vi "FreqC.Open Session.vi"(8 "error In":errorcluster, 11 "VISA resource name":refnum<visa-resource-name>) -> (0 "error out":errorcluster, 3 "FreqC Session out":T1)   [LabVIEW 2018]
uses:
  typedefs/FreqC.Session.ctl
  <instrlib>/Agilent 532XX Series/Public/Configure/Configure Channel (Basic).vi
  <instrlib>/Agilent 532XX Series/Public/Configure/Configure Channel (Voltage Range).vi
  <instrlib>/Agilent 532XX Series/Public/Configure/Configure Channel (Slop).vi
  <instrlib>/Agilent 532XX Series/Public/Configure/Configure Channel (Threshold Voltage).vi
  <instrlib>/Agilent 532XX Series/Public/Configure/Measurement/Configure Measurement (Totalize Timed).vi
  <instrlib>/Agilent 532XX Series/Agilent 532XX Series.lvlib
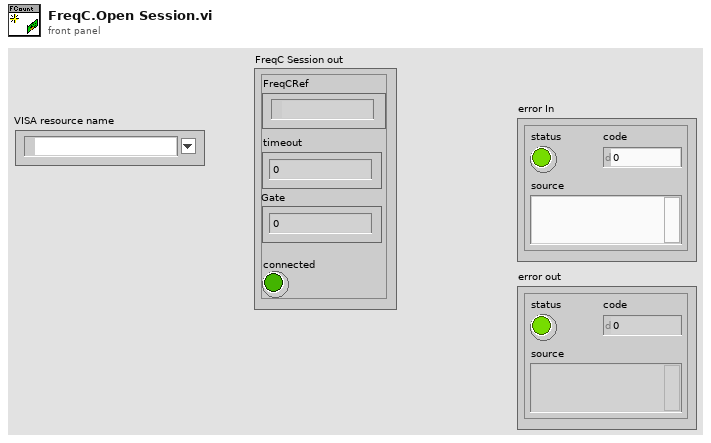
[diagram p1: front panel]
types:
  T1 = typedef "FreqC.Session.ctl" = cluster{"FreqCRef":refnum<visa-resource-name>, "timeout":dbl, "Gate":dbl, "connected":bool}
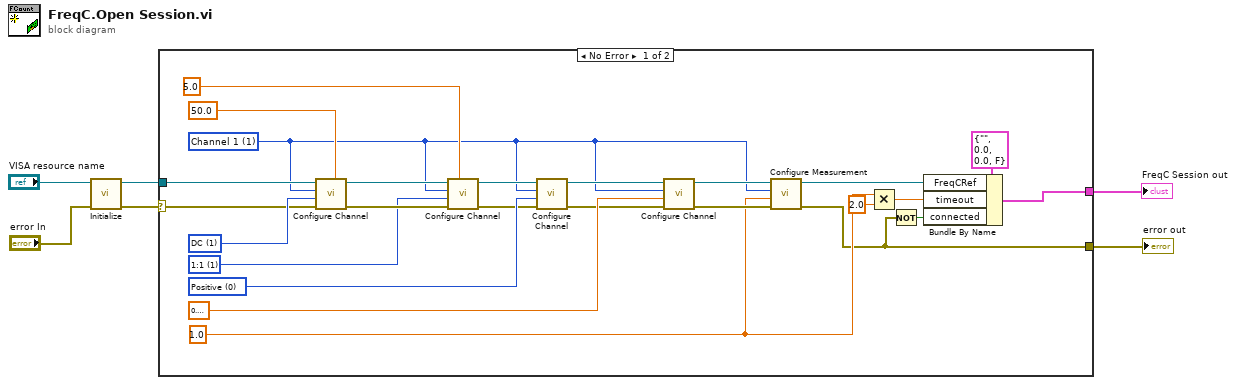
[diagram p0: block diagram]
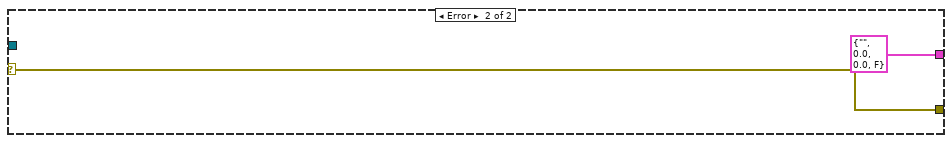
[diagram p2: hidden frame]
diagram:
  n1 = call <instrlib>:"Initialize.vi"("error in (no error)"="error In", "VISA resource name"="VISA resource name") -> ("error out"=w1:errorcluster, "VISA resource name out"=w6:refnum<visa-resource-name>)  [unwired: 8 in]
  n2 = case shown="No Error" w1 {
    selector: w1 -> [w12 w33]
    tunnel: w6 -> [w31 _]
    tunnel: [w7 w33] -> w3
    tunnel: [w13 T1 {"FreqCRef"="", "timeout"=0.0, "Gate"=0.0, "connected"=FALSE} ("FreqC.Session")] -> w2
    frame No Error {
      w11 = 1.0 ("Timed Totalize (0.1 s)")
      w24 = 0 items=["Positive", "Negative"] ("Active Edge (1: Negative)")
      w26 = 1 items=["1:1"=1, "10:1"=10] ("Probe Factor ( 1:1)")
      w29 = 50.0 items=["50"=50.0, "1E+6"=1000000.0] ("Impedance (1E+6 Ohm)")
      w30 = 1 items=["AC", "DC"] ("Coupling (0: AC)")
      w17 = 1 items=["Channel 1"=1, "Channel 2"=2] ("Channel (1: Channel 1)")
      n3 = call-poly <instrlib>:"Configure Channel.vi"("Impedance (1E+6 Ohm)"=w29, "error in (no error)"=w12, "Coupling (0: AC)"=w30, "Channel (1: Channel 1)"=w17, "VISA resource name"=w31) -> ("error out"=w28:errorcluster, "VISA resource name out"=w27:refnum<visa-resource-name>)  [unwired: 5 in]
      n4 = call-poly <instrlib>:"Configure Channel.vi"("Voltage Range (5V)"=5.0, "error in (no error)"=w28, "Probe Factor ( 1:1)"=w26, "Channel (1: Channel 1)"=w17, "VISA resource name"=w27) -> ("error out"=w22:errorcluster, "VISA resource name out"=w23:refnum<visa-resource-name>)  [unwired: 5 in]
      n5 = call-poly <instrlib>:"Configure Channel.vi"("error in (no error)"=w22, "Active Edge (1: Negative)"=w24, "Channel (1: Channel 1)"=w17, "VISA resource name"=w23) -> ("error out"=w19:errorcluster, "VISA resource name out"=w20:refnum<visa-resource-name>)  [unwired: 6 in]
      n6 = call-poly <instrlib>:"Configure Channel.vi"("error in (no error)"=w19, "Threshold Voltage (0 V)"=0.30000000000000004, "Channel (1: Channel 1)"=w17, "VISA resource name"=w20) -> ("error out"=w16:errorcluster, "VISA resource name out"=w18:refnum<visa-resource-name>)  [unwired: 6 in]
      n7 = call-poly <instrlib>:"Configure Measurement.vi"("error in (no error)"=w16, "Timed Totalize (0.1 s)"=w11, "Channel (1: Channel 1)"=w17, "VISA resource name"=w18) -> ("error out"=w7:errorcluster, "VISA resource name out"=w14:refnum<visa-resource-name>)  [unwired: 6 in]
      n8 = Multiply(x=w11, y=2.0) -> (x*y=w10:dbl)
      n9 = Not(x=w7) -> (.not. x?=w8:bool)
      n10 = Bundle By Name(cluster=T1 {"FreqCRef"="", "timeout"=0.0, "Gate"=0.0, "connected"=FALSE} ("FreqC.Session"), "FreqCRef"=w14, "timeout"=w10, "connected"=w8) -> (w13:T1)
    }
    frame Error {
    }
  }
  "error out" <- w3
  "FreqC Session out" <- w2
